vi "Order Rectangle & Median Coordinates.vi"(9 "EF":i32[](array[numeric]), 11 "ABCD":i32[](array[numeric])) -> (1 "Median":i32[](array[numeric]), 3 "Rectangle":i32[](array[numeric]))   [LabVIEW 2021, in "Image.lvlib"]
uses:
  Image.lvlib
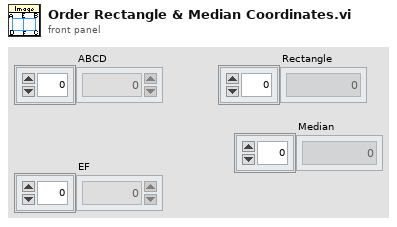
[diagram p1: front panel]
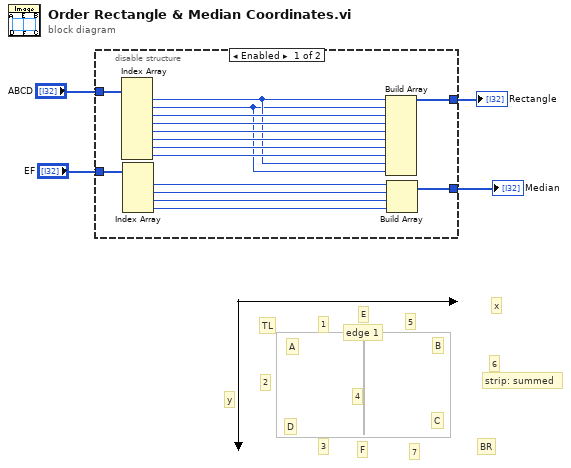
[diagram p0: block diagram]
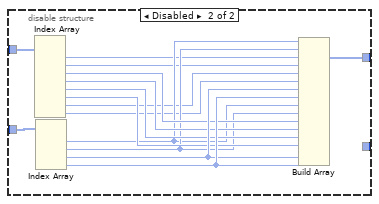
[diagram p2: hidden frame]
diagram:
  # "7"
  # "6"
  # "5"
  # "4"
  # "3"
  # "2"
  # "1"
  # "F"
  # "E"
  # "strip: summed"
  # "D"
  # "C"
  # "B"
  # "A"
  # "edge 1"
  # "x"
  # "y"
  # "BR"
  # "TL"
  n1 = disable-structure shown="Enabled" {
    disable-tunnel: "EF" -> [w20 w23]
    disable-tunnel: [w8 w22] -> w3
    disable-tunnel: "ABCD" -> [w19 w21]
    disable-tunnel: [w7 _] -> w1
    frame Enabled {
      n2 = Index Array(array=w19) -> (element #1=w12:i32, element #2=w11:i32, element #3=w18:i32, element #4=w17:i32, element #5=w16:i32, element #6=w15:i32, element #7=w14:i32, element #8=w13:i32)  [unwired: 8 in]
      n3 = Index Array(array=w20) -> (element #1=w10:i32, element #2=w9:i32, element #3=w6:i32, element #4=w5:i32)  [unwired: 4 in]
      n4 = Build Array(w12, w11, w18, w17, w16, w15, w14, w13, w12, w11) -> (w8:i32[])
      n5 = Build Array(w10, w9, w6, w5) -> (w7:i32[])
    }
    frame Disabled {
      n6 = Index Array(array=w21) -> (element #1=w24:i32, element #2=w25:i32, element #3=w30:i32, element #4=w31:i32, element #5=w32:i32, element #6=w33:i32, element #7=w26:i32, element #8=w27:i32)  [unwired: 8 in]
      n7 = Index Array(array=w23) -> (element #1=w28:i32, element #2=w29:i32, element #3=w34:i32, element #4=w35:i32)  [unwired: 4 in]
      n8 = Build Array(w28, w29, w24, w25, w26, w27, w34, w35, w28, w29, w30, w31, w32, w33, w34, w35) -> (w22:i32[])
    }
  }
  "Rectangle" <- w3
  "Median" <- w1
